vi "Plot Graph.vi"(7 "path to PNG file":path, 10 "Log Data":string[][](array[string]), 11 "Indexes":i32[](array[numeric])) -> (3 "Plot Path":path)   [LabVIEW 2014]
panel:
  out "Pressure Plot":cluster{timestamp[], dbl[]}[](graph)
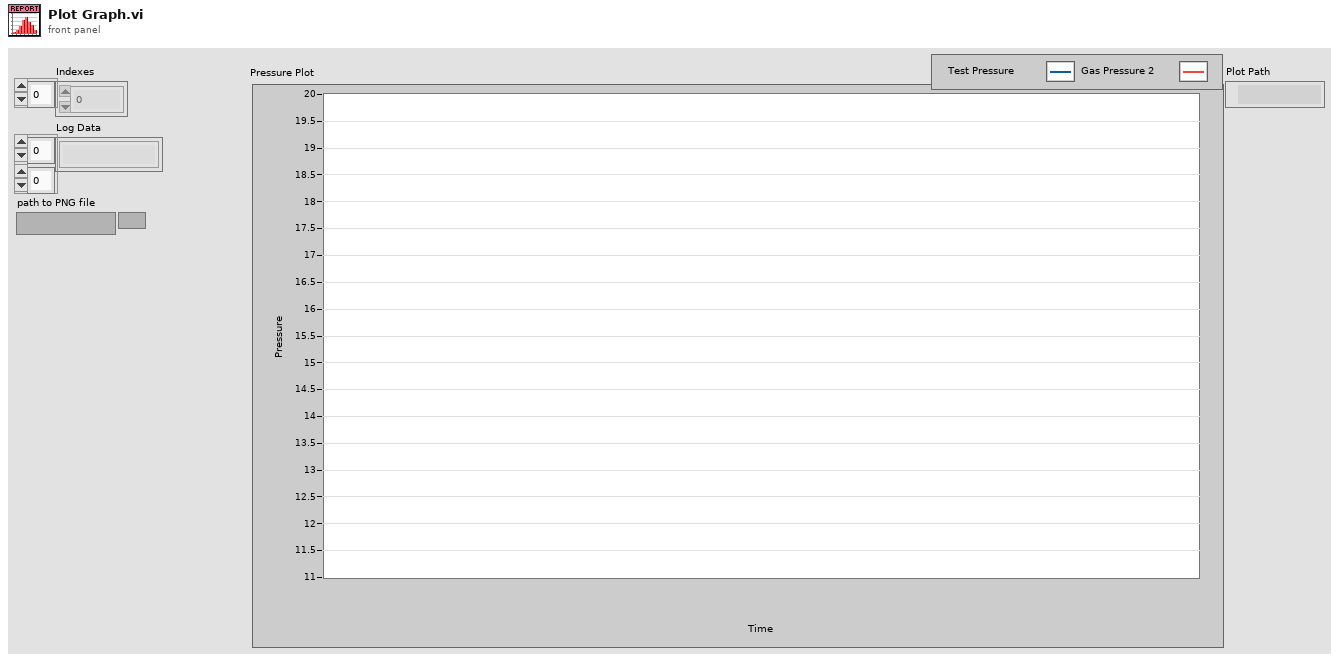
[diagram p1: front panel]
types:
  T1 = typedef "imagedata.ctl" = cluster{"image type":i32, "image depth":i32, "image":u8[], "mask":u8[], "colors":u32[], "Rectangle":cluster{"left":i16, "top":i16, "right":i16, "bottom":i16}}
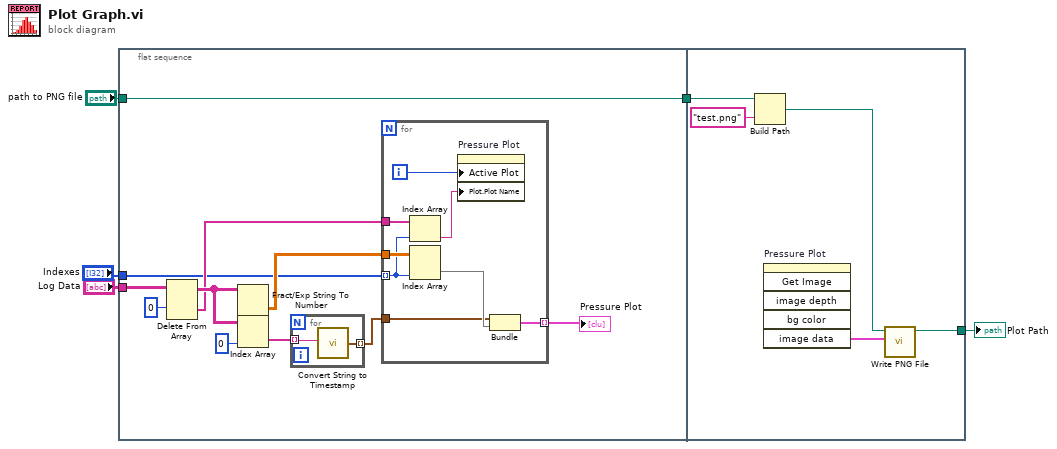
[diagram p0: block diagram]
diagram:
  n1 = flat-sequence {
    tunnel: "Indexes" -> [w8]
    tunnel: "Log Data" -> [w7]
    tunnel: [w6] -> w3
    tunnel: "path to PNG file" -> [w6]
    tunnel: w3 -> [w30]
    tunnel: [w27] -> w1
    frame #0 {
      n2 = Delete From Array(array=w7, index (row)=0) -> (deleted portion=w9:string[], array with subset deleted=w13:string[][])  [unwired: 2 in]
      n3 = Fract/Exp String To Number(string=w13) -> (number=w15:dbl[][])  [unwired: 3 in, 1 out]
      n4 = Index Array(array=w13, index (col)=0 ("disabled index (col)")) -> (element=w11:string[])  [unwired: 1 in]
      n5 = for {
        tunnel: w11 -> [w18] mode=indexing
        tunnel: [w17] -> w10 mode=indexing
        n6 = call "Convert String to Timestamp.vi"("date/time string"=w18) -> ("Resulting Time Stamp"=w17:timestamp)
      }
      n7 = for {
        tunnel: w8 -> [w20] mode=indexing
        tunnel: [w24] -> w14 mode=indexing
        tunnel: w10 -> [w23]
        tunnel: w9 -> [w21]
        tunnel: w15 -> [w26]
        i -> [w22]
        n8 = Index Array(array=w21, index=w20) -> (element=w19:string)
        n9 = Index Array(array=w26, index (col)=w20) -> (element=w25:dbl[])  [unwired: 1 in]
        n10 = property on="Pressure Plot" class="XYGraph (strict)"("Active Plot"=w22, "Plot.Plot Name"=w19) -> ()  [unwired: 2 in, 2 out]
        n11 = Bundle(w23, w25) -> (w24:cluster{timestamp[], dbl[]})  [unwired: 1 in]
      }
      "Pressure Plot" <- w14
    }
    frame #1 {
      n12 = Build Path(base path=w30, name or relative path="test.png") -> (appended path=w28:path)
      n13 = invoke on="Pressure Plot" class="XYGraph (strict)" method="Get Image"() -> ("image data"=w31:T1)  [unwired: 6 in, 5 out]
      n14 = call <vilib>:"Write PNG File.vi"("image data"=w31, "path to PNG file"=w28) -> ("path"=w27:path)  [unwired: 8 in, 1 out]
    }
  }
  "Plot Path" <- w1
